vi "Stop.vi"(8 "error in (no error)":errorcluster, 11 "Thermometer DAQmx in":refnum<class "Thermometer DAQmx.lvclass">) -> (0 "error out":errorcluster, 3 "Thermometer DAQmx out":refnum<class "Thermometer DAQmx.lvclass">)   [LabVIEW 2023, in "Thermometer.lvlib" / "Thermometer DAQmx.lvlib" / "Thermometer DAQmx.lvclass"]
uses:
  Thermometer DAQmx.lvclass
  Thermometer DAQmx.lvclass/Thermometer DAQmx.ctl
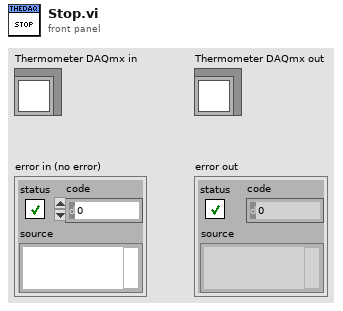
[diagram p1: front panel]
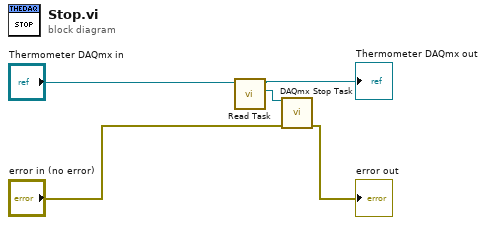
[diagram p0: block diagram]
diagram:
  n1 = call-dynamic "Read Task.vi"("Thermometer DAQmx in"="Thermometer DAQmx in") -> ("Task"=w4:refnum<k21>, "Thermometer DAQmx out"=→"Thermometer DAQmx out":refnum<class "Thermometer DAQmx.lvclass">)  [unwired: 8 in, 1 out]
  n2 = call <vilib>:"DAQmx Stop Task.vi"("task/channels in"=w4, "error in"="error in (no error)") -> ("error out"=→"error out":errorcluster)  [unwired: 12 in, 1 out]
